vi "Initialize.vi"(8 "error in":errorcluster, 11 "Light Stack in":refnum<class "Light Stack.lvclass">) -> (0 "error out":errorcluster, 3 "Light Stack out":refnum<class "Light Stack.lvclass">)   [LabVIEW 2018, in "Light Stack.lvlib" / "Light Stack.lvclass"]
uses:
  Light Stack.lvclass
  Custom Controls/Light Select.ctl
  Custom Controls/Light Mode.ctl
  Light Stack.lvclass/Light Stack.ctl
  Light Stack.lvlib
panel:
  in  "Light Select":T1
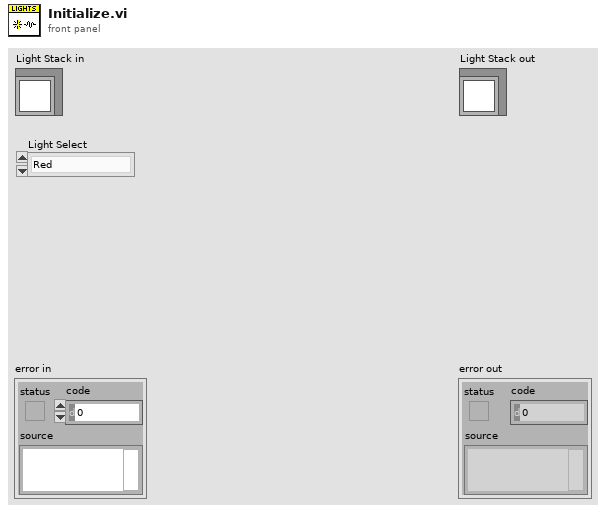
[diagram p1: front panel]
types:
  T1 = typedef "Light Stack.lvlib/Light Select.ctl" = enum16{"Red", "Amber", "Green", "Blue"}
  T2 = typedef "Light Stack.lvlib/Light Mode.ctl" = enum16{"OFF", "ON", "BLINK"}
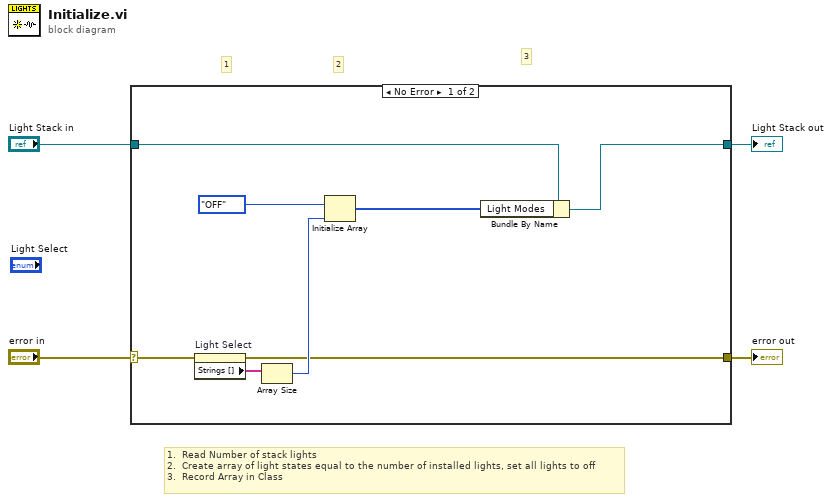
[diagram p0: block diagram]
diagram:
  # "3"
  # "2"
  # "1"
  # "1.  Read Number of stack lights\n2.  Create array of light states equal to the number of installed lights, set all lights to off\n3.  Record Array in Class"
  n1 = case shown="No Error" "error in" {
    selector: "error in" -> [w6 w14]
    tunnel: [w5 w14] -> w3
    tunnel: [w8 w13] -> w1
    tunnel: "Light Stack in" -> [w12 w13]
    frame No Error {
      n2 = property on="Light Select" class="Enum (strict)"(error in=w6) -> (error out=w5:errorcluster, "Strings []"=w11:string[])  [unwired: 1 in, 1 out]
      n3 = Array Size(array=w11) -> (size(s)=w10:i32)
      n4 = Initialize Array(Light_Mode."OFF" ("Light Mode"), w10) -> (w7:T2[])
      n5 = Bundle By Name(cluster=w12, "Light Modes"=w7) -> (w8:refnum<class "Light Stack.lvclass">)
    }
    frame Error {
    }
  }
  "error out" <- w3
  "Light Stack out" <- w1
